vi "AdaptToInputs.vi"(0 "XRef":T12, 1 "Term Types":T10, 2 "State In":T1 {"BlockNodeState"."Draw Style" items=["FunctionBlock", "ExpressVI", "Variable", "Elemental I/O", "32x32 Icon", "FunctionBlockCompact"]; "BlockNodeState"."Terminal Data"."Terminal Flags" format="%.0b"}) -> (14 "Reply":T8, 15 "State Out":T1 {"BlockNodeState"."Draw Style" items=["FunctionBlock", "ExpressVI", "Variable", "Elemental I/O", "32x32 Icon", "FunctionBlockCompact"]; "BlockNodeState"."Terminal Data"."Terminal Flags" format="%.0b"})   [LabVIEW 2020, in "NI_ExpressFull.lvlib" / "ExpressSpectralMeasurementsBlockNode.xnode"]
uses:
  <vilib>/express/express analysis/Spectral/XNode/ExpressSpectralMeasurementsBlockNode.xnode
  <vilib>/XNodeSupport/XNodeXNodeRef.ctl
  <vilib>/XNodeSupport/NI_XNodeSupport.lvlib
  <vilib>/XNodeSupport/XNodeString.ctl
  <vilib>/XNodeSupport/XNodeType.ctl
  <vilib>/XNodeSupport/XNodeTermTypeIDPair.ctl
  <vilib>/XNodeSupport/XNodeTermTypeIDPairs.ctl
  <vilib>/XNodeSupport/XNodeStringArray.ctl
  <vilib>/picture/picture.llb/imagedata.ctl
  <vilib>/BlockNodeSupport/BlockNodeState.ctl
  <vilib>/express/express analysis/Spectral/XNode/State.ctl
  <vilib>/express/express shared/XNodes/controls/ExpressState.ctl
  <vilib>/BlockNodeSupport/TerminalData.ctl
  <vilib>/express/express shared/XNodes/controls/ExpressTerminalInfo.ctl
panel:
  in  "[Phase]":cluster{"f0":dbl, "df":dbl, "phase":dbl[]}[](graph)
  in  "Measurement Output":cluster{"f0":dbl, "df":dbl, "magnitude":dbl[]}(graph)
  in  "Phase":cluster{"f0":dbl, "df":dbl, "phase":dbl[]}(graph)
  in  "[Measurement Output]":cluster{"f0":dbl, "df":dbl, "magnitude":dbl[]}[](graph)
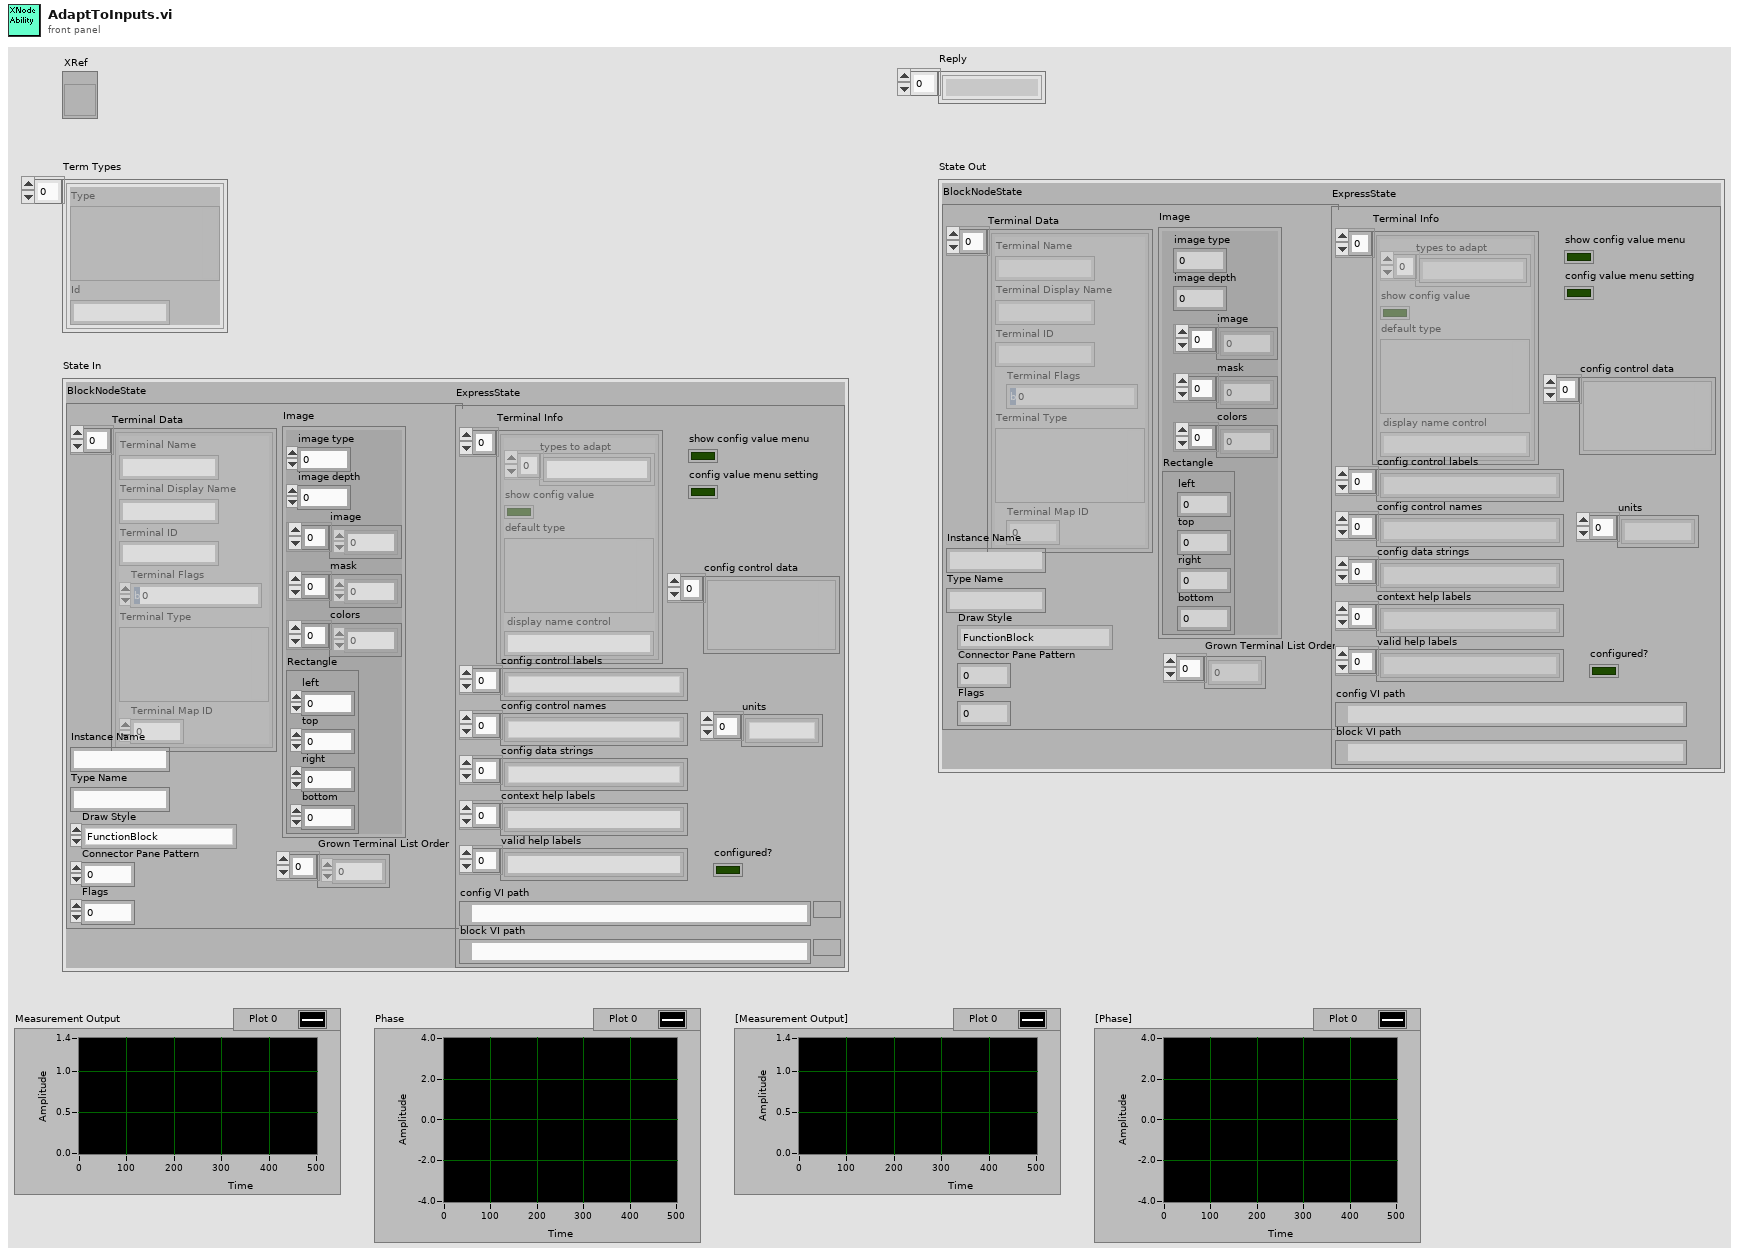
[diagram p1: front panel]
types:
  T1 = typedef "NI_ExpressFull.lvlib/ExpressSpectralMeasurementsBlockNode.xnode/State.ctl" = cluster{"BlockNodeState":T2, "ExpressState":T5}
  T2 = typedef "BlockNodeState.ctl" = cluster{"Terminal Data":T3[], "Instance Name":string, "Type Name":string, "Draw Style":i32, "Connector Pane Pattern":i32, "Flags":i32, "Grown Terminal List Order":i32[], "Image":T4}
  T3 = typedef "TerminalData.ctl" = cluster{"Terminal Name":string, "Terminal Display Name":string, "Terminal ID":string, "Terminal Flags":i32, "Terminal Type":variant, "Terminal Map ID":i32}
  T4 = typedef "imagedata.ctl" = cluster{"image type":i32, "image depth":i32, "image":u8[], "mask":u8[], "colors":u32[], "Rectangle":cluster{"left":i16, "top":i16, "right":i16, "bottom":i16}}
  T5 = typedef "ExpressState.ctl" = cluster{"Terminal Info":T6, "config control names":string[], "config data strings":string[], "config control data":variant[], "units":string[], "configured?":bool, "config VI path":path, "block VI path":path, "config control labels":string[], "show config value menu":bool, "config value menu setting":bool, "context help labels":string[], "valid help labels":string[]}
  T6 = typedef "ExpressTerminalInfo.ctl" = cluster{"types to adapt":string[], "show config value":bool, "default type":T7, "display name control":string}[]
  T7 = typedef "NI_XNodeSupport.lvlib/XNodeType.ctl" = variant
  T8 = typedef "NI_XNodeSupport.lvlib/XNodeStringArray.ctl" = T9[]
  T9 = typedef "NI_XNodeSupport.lvlib/XNodeString.ctl" = string
  T10 = typedef "NI_XNodeSupport.lvlib/XNodeTermTypeIDPairs.ctl" = T11[]
  T11 = typedef "NI_XNodeSupport.lvlib/XNodeTermTypeIDPair.ctl" = cluster{"Type":T7, "Id":T9}
  T12 = typedef "NI_XNodeSupport.lvlib/XNodeXNodeRef.ctl" = refnum<vi>
  T13 = typedef "ExpressBlockNodeState.ctl" = cluster{"BlockNodeState":T2, "ExpressState":T5}
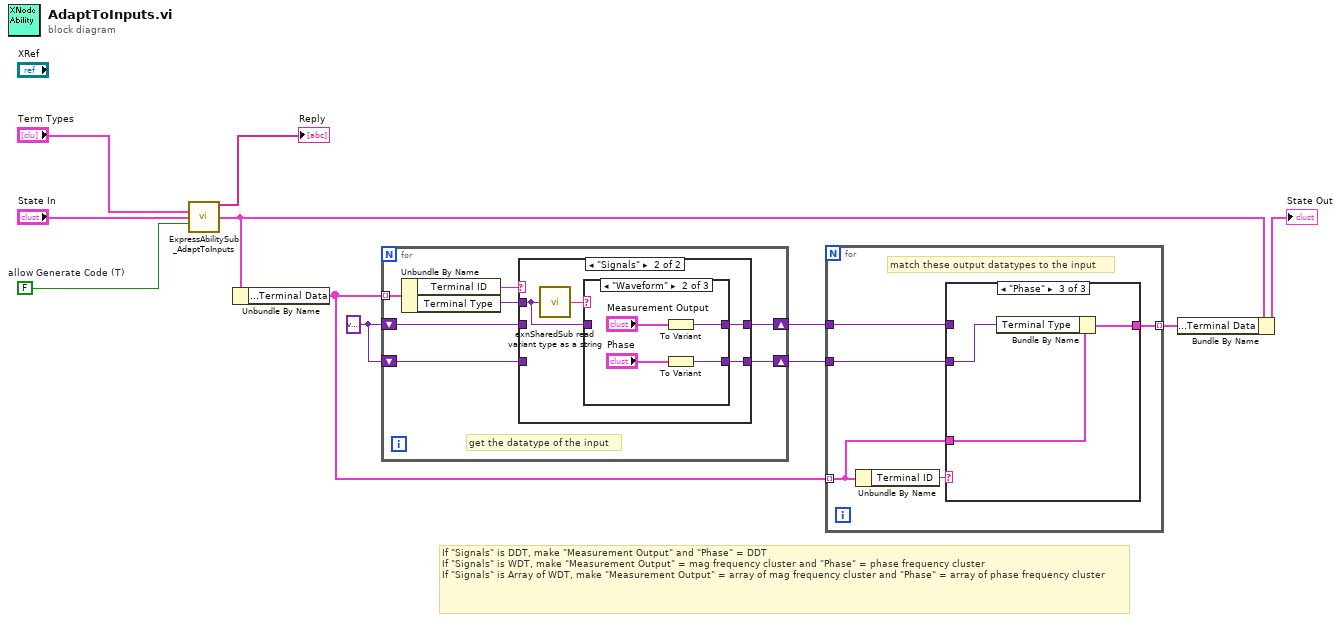
[diagram p0: block diagram]
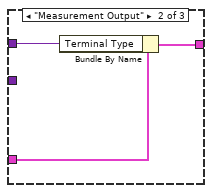
[diagram p3: hidden frame]
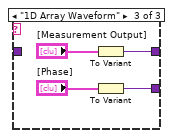
[diagram p6: hidden frame]
diagram:
  w2 = variant ("Terminal Type")
  w8 = FALSE  # allow Generate Code (T)
  # "If \"Signals\" is DDT, make \"Measurement Output\" and \"Phase\" = DDT\nIf \"Signals\" is WDT, make \"Measurement Output\" = mag frequency cluster and \"Phase\" = phase frequency cluster\nIf \"Signals\" is Array of WDT, make \"Measurement Output\" = array of mag frequency cluster and \"Phase\" = array of phase frequency cluster"
  n1 = call <vilib>:"ExpressAbilitySub_AdaptToInputs.vi"("Term Types"="Term Types", "ExpressBlockNodeState In"="State In", "allow Generate Code (T)"=w8) -> ("Reply"=→"Reply":string[], "ExpressBlockNodeState Out"=w5:T13)  [unwired: 11 in]
  n2 = Unbundle By Name(w5) -> ("BlockNodeState.Terminal Data"=w7:T3[])
  n3 = for {
    tunnel: w7 -> [w18] mode=indexing
    shift-right: [w16] -> w6
    shift-left: w2 -> [w14]
    shift-right: [w12] -> w1
    shift-left: w2 -> [w13]
    # "get the datatype of the input"
    n4 = Unbundle By Name(w18) -> ("Terminal ID"=w17:string, "Terminal Type"=w15:variant)
    n5 = case shown="\"Signals\"" w17 {
      tunnel: [w20 w23] -> w16
      tunnel: w15 -> [_ w21]
      tunnel: w14 -> [w20 _]
      tunnel: w13 -> [w19 _]
      tunnel: [w19 w22] -> w12
      frame Default {
      }
      frame "Signals" {
        n6 = call <vilib>:"exnSharedSub read variant type as a string.vi"("Variant"=w21) -> ("type as string"=w24:string)  [unwired: 14 in]
        n7 = case shown="\"Waveform\"" w24 {
          tunnel: [w25 w27 w32] -> w23
          tunnel: [w25 w29 w33] -> w22
          tunnel: w21 -> [w25 _ _]
          frame "ExpressData", Default {
          }
          frame "Waveform" {
            n8 = To Variant(anything="Measurement Output") -> (Variant=w27:variant)
            n9 = To Variant(anything="Phase") -> (Variant=w29:variant)
          }
          frame "1D Array Waveform" {
            n10 = To Variant(anything="[Measurement Output]") -> (Variant=w32:variant)
            n11 = To Variant(anything="[Phase]") -> (Variant=w33:variant)
          }
        }
      }
    }
  }
  n12 = for {
    tunnel: w7 -> [w37] mode=indexing
    tunnel: w6 -> [w36]
    tunnel: [w35] -> w3 mode=indexing
    tunnel: w1 -> [w34]
    # "match these output datatypes to the input"
    n13 = Unbundle By Name(w37) -> ("Terminal ID"=w38:string)
    n14 = case shown="\"Phase\"" w38 {
      tunnel: w37 -> [w39 w42 w45]
      tunnel: w36 -> [_ w41 _]
      tunnel: [w39 w40 w44] -> w35
      tunnel: w34 -> [_ _ w43]
      frame Default {
      }
      frame "Measurement Output" {
        n15 = Bundle By Name(cluster=w42, "Terminal Type"=w41) -> (w40:T3)
      }
      frame "Phase" {
        n16 = Bundle By Name(cluster=w45, "Terminal Type"=w43) -> (w44:T3)
      }
    }
  }
  n17 = Bundle By Name(cluster=w5, "BlockNodeState.Terminal Data"=w3) -> (→"State Out":T13)
